vi "貪食蛇01.vi"() -> ()   [LabVIEW 2021]
uses:
  <vilib>/Utility/inputDevices.llb/keyboardAcquire.vi
  <vilib>/Utility/inputDevices.llb/closeKeyboard.vi
panel:
  out "第三次果實":dbl
  out "第二次果實":dbl
  out "第一次果實":dbl
  out "達成成就":string
  in  "OK Button":bool
  out "String":string
  in  "reset":bool
  out "時間(秒)":dbl
  out "計分板":dbl
  in  "stop":bool
  out "Array":bool[][](array[boolean])
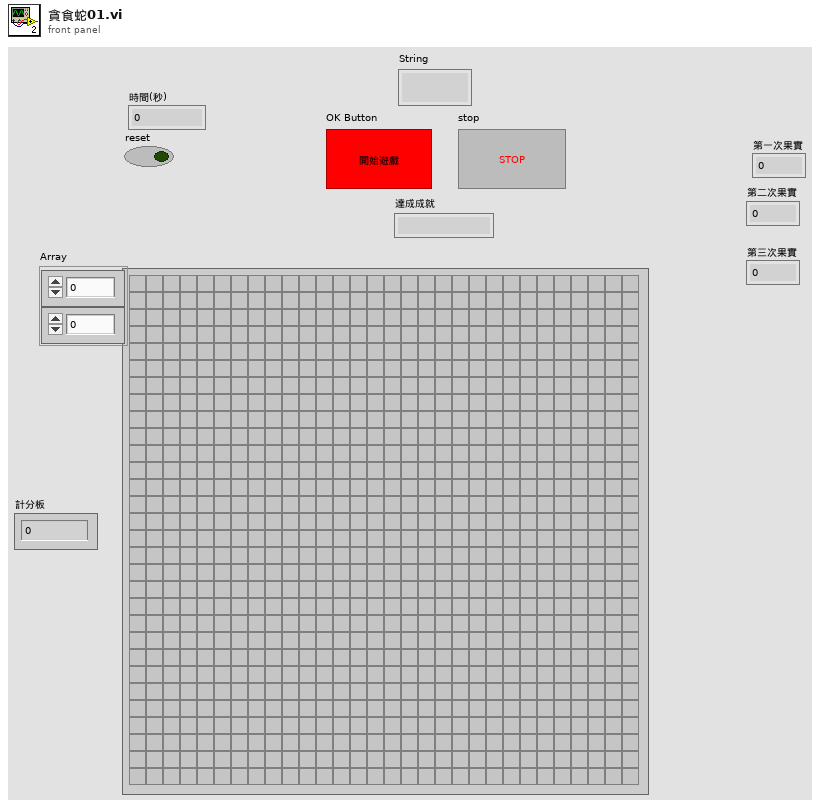
[diagram p1: front panel]
types:
  T1 = enum16{"0", "1", "2", "3", "4", "5", "6", "7", "8", "9", "A", "B", "C", "D", "E", "F", "G", "H", "I", "J", "K", "L", "M", "N", "O", "P", "Q", "R", "S", "T", "U", "V", "W", "X", "Y", "Z", "F1", "F2", "F3", "F4", "F5", "F6", "F7", "F8", "F9", "F10", "F11", "F12", "F13", "F14", "F15", "ADD", "BACK", "BACKSLASH", "CAPITAL", "COMMA", "DECIMAL", "DELETE", "DIVIDE", "DOWN", "END", "EQUALS", "ESCAPE", "GRAVE (`)", "HOME", "INSERT", "LBRACKET", "LCONTROL", "LEFT", "L ALT", "LSHIFT", "LWIN", "MINUS", "MULTIPLY", "NEXT", "NUMLOCK", "NUMPAD_0", "NUMPAD_1", "NUMPAD_2", "NUMPAD_3", "NUMPAD_4", "NUMPAD_5", "NUMPAD_6", "NUMPAD_7", "NUMPAD_8", "NUMPAD_9", "PAUSE", "PERIOD", "PRIOR (PG UP)", "RBRACKET", "RCONTROL", "RETURN", "RIGHT", "R ALT", "RSHIFT", "RWIN", "SCROLL", "SEMICOLON", "SLASH", "SPACE", "SUBTRACT", "TAB", "UP", "ENTER (num pad)", "' (quote)"}[]
  T2 = enum16{"0", "1", "2", "3", "4", "5", "6", "7", "8", "9", "A", "B", "C", "D", "E", "F", "G", "H", "I", "J", "K", "L", "M", "N", "O", "P", "Q", "R", "S", "T", "U", "V", "W", "X", "Y", "Z", "F1", "F2", "F3", "F4", "F5", "F6", "F7", "F8", "F9", "F10", "F11", "F12", "F13", "F14", "F15", "ADD", "BACK", "BACKSLASH", "CAPITAL", "COMMA", "DECIMAL", "DELETE", "DIVIDE", "DOWN", "END", "EQUALS", "ESCAPE", "GRAVE (`)", "HOME", "INSERT", "LBRACKET", "LCONTROL", "LEFT", "L ALT", "LSHIFT", "LWIN", "MINUS", "MULTIPLY", "NEXT", "NUMLOCK", "NUMPAD_0", "NUMPAD_1", "NUMPAD_2", "NUMPAD_3", "NUMPAD_4", "NUMPAD_5", "NUMPAD_6", "NUMPAD_7", "NUMPAD_8", "NUMPAD_9", "PAUSE", "PERIOD", "PRIOR (PG UP)", "RBRACKET", "RCONTROL", "RETURN", "RIGHT", "R ALT", "RSHIFT", "RWIN", "SCROLL", "SEMICOLON", "SLASH", "SPACE", "SUBTRACT", "TAB", "UP", "ENTER (num pad)", "' (quote)"}
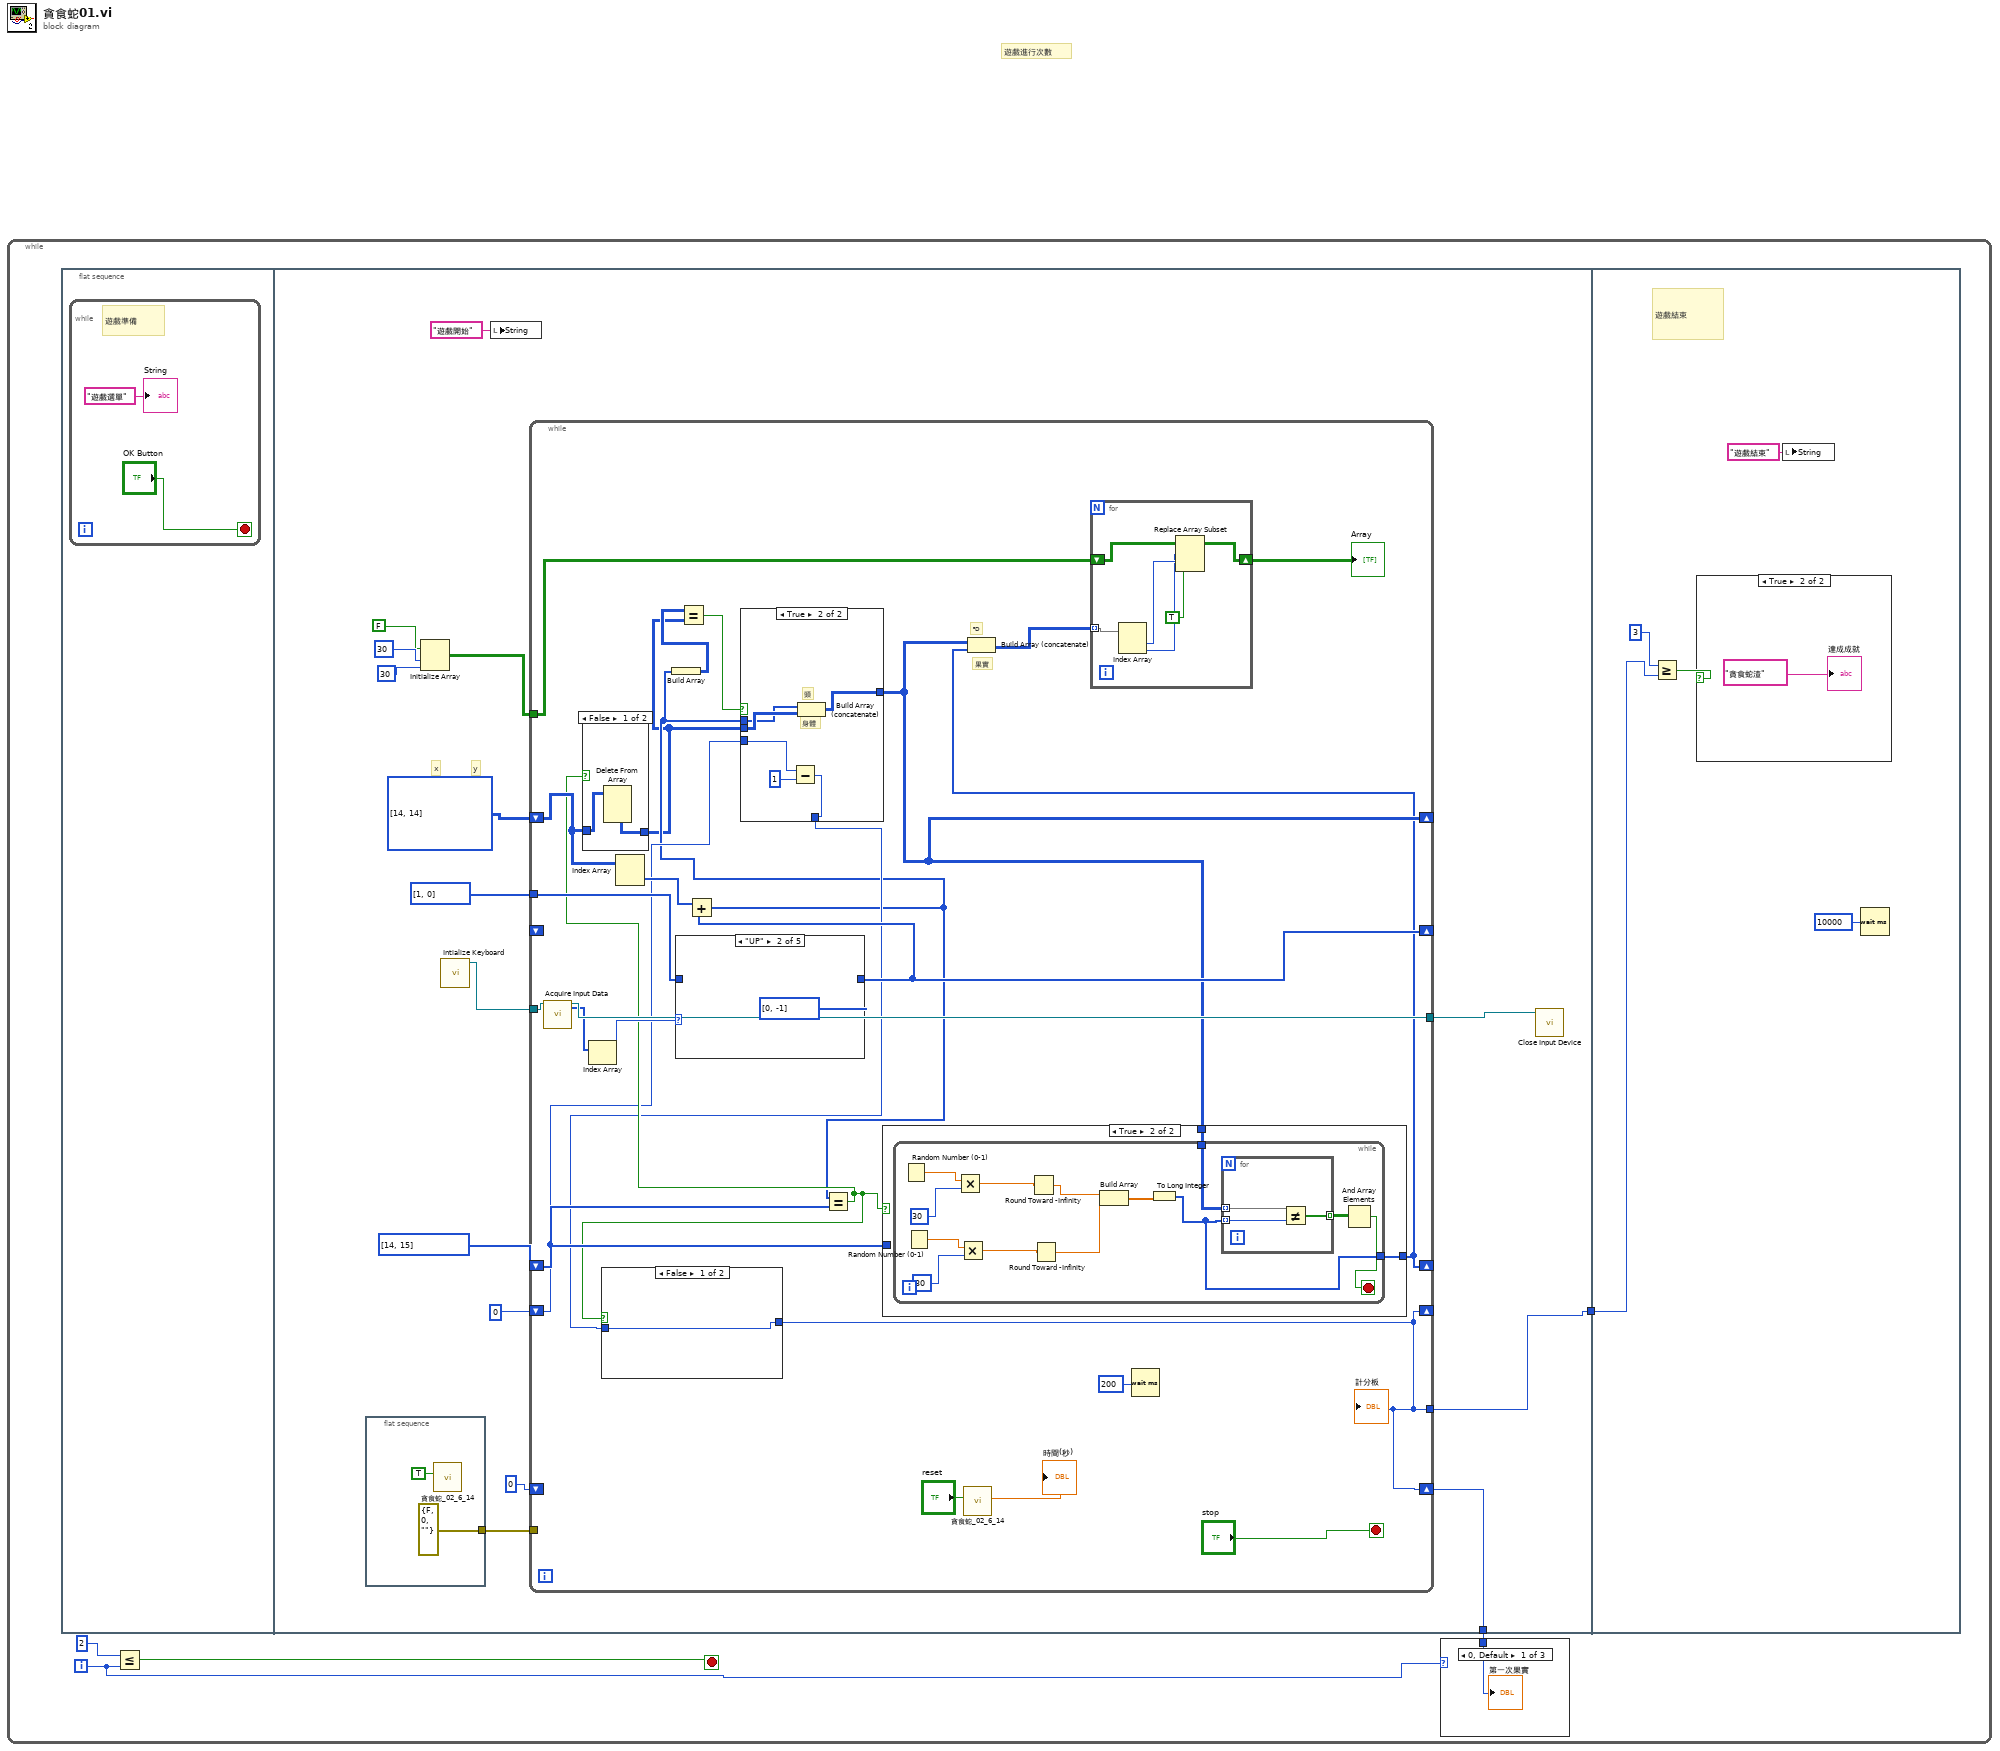
[diagram p0: block diagram]
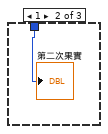
[diagram p2: hidden frame]
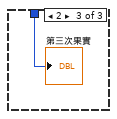
[diagram p3: hidden frame]
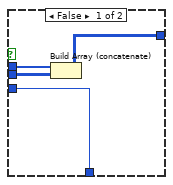
[diagram p4: hidden frame]
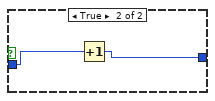
[diagram p5: hidden frame]
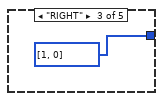
[diagram p9: hidden frame]
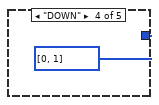
[diagram p10: hidden frame]
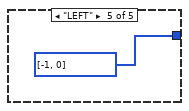
[diagram p11: hidden frame]
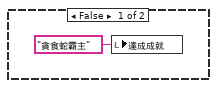
[diagram p12: hidden frame]
diagram:
  # "遊戲進行次數"
  n1 = while {
    i -> [w2]
    stop <- w3 stop-if-true
    n2 = flat-sequence {
      tunnel: [w13] -> w5
      tunnel: [w11] -> w1
      tunnel: w5 -> [w102]
      frame #0 {
        n3 = while {
          stop <- "OK Button" stop-if-true
          # "遊戲準備"
          "String" <- "遊戲選單" ("String")
        }
      }
      frame #1 {
        # "y"
        # "x"
        n4 = flat-sequence {
          tunnel: [errorcluster {"status"=FALSE, "code"=0, "source"=""} ("error constant")] -> w15
          frame #0 {
            n5 = call "貪食蛇_02_6_14.vi"("reset"=TRUE) -> ()  [unwired: 10 in, 1 out]
          }
        }
        n6 = Initialize Array(FALSE, 30, 30) -> (w22:bool[][])
        n7 = call <vilib>:"Intialize Keyboard.vi"() -> ("device ID"=w21:refnum<k1>)  [unwired: 10 in, 1 out]
        n8 = local write "String"("遊戲開始" ("String")) -> ()
        n9 = while {
          tunnel: w22 -> [w50]
          tunnel: w21 -> [w52]
          tunnel: [w51] -> w20
          shift-right: [w43] -> _
          shift-left: i32[][] [[14, 14]] -> [w44]
          shift-right: [w45] -> _
          shift-left: _ -> [_]
          tunnel: i32[] [1, 0] -> [w47]
          shift-right: [w40] -> _
          shift-left: i32[] [14, 15] -> [w42]
          shift-right: [w34] -> _
          shift-left: 0 -> [w33]
          tunnel: w15 -> [_]
          tunnel: [w34] -> w13
          shift-right: [w34] -> w11
          shift-left: 0 -> [_]
          stop <- "stop" stop-if-true
          # "果實"
          # "³D"
          n10 = call-poly <vilib>:"Acquire Input Data.vi"("device ID"=w52) -> ("device ID"=w51:refnum<k1>, "keys pressed"=w37:T1)  [unwired: 16 in, 1 out]
          n11 = Index Array(array=w37) -> (element=w48:T2)  [unwired: 1 in]
          n12 = Index Array(array=w44) -> (element=w46:i32[])  [unwired: 2 in]
          n13 = case shown="\"UP\"" w48 {
            tunnel: w47 -> [w89 _ _ _ _]
            tunnel: [w89 i32[] [0, -1] i32[] [1, 0] i32[] [0, 1] i32[] [-1, 0]] -> w45
            frame "0", Default {
            }
            frame "UP" {
            }
            frame "RIGHT" {
            }
            frame "DOWN" {
            }
            frame "LEFT" {
            }
          }
          n14 = Add(x=w46, y=w45) -> (x+y=w30:i32[])
          n15 = Build Array(w30) -> (w29:i32[][])
          n16 = Equal?(x=w30, y=w42) -> (x = y?=w39:bool)
          n17 = case shown="False" w39 {
            tunnel: [w87 w88] -> w28
            tunnel: w44 -> [w86 w88]
            frame False {
              n18 = Delete From Array(array=w86) -> (array with subset deleted=w87:i32[][])  [unwired: 3 in, 1 out]
            }
            frame True {
            }
          }
          n19 = Equal?(x=w29, y=w28) -> (x = y?=w31:bool)
          n20 = case shown="True" w31 {
            tunnel: [w57 w61] -> w43
            tunnel: w30 -> [w56 w62]
            tunnel: w28 -> [w55 w63]
            tunnel: w33 -> [w54 w59]
            tunnel: [w54 w58] -> w32
            frame False {
              n21 = Build Array (concatenate)(w56, w55) -> (w57:i32[][])
            }
            frame True {
              # "身體"
              # "頭"
              n22 = Subtract(x=w59, y=1) -> (x-y=w58:i32)
              n23 = Build Array (concatenate)(w62, w63) -> (w61:i32[][])
            }
          }
          n24 = case shown="False" w39 {
            tunnel: w32 -> [w64 w66]
            tunnel: [w64 w65] -> w34
            frame False {
            }
            frame True {
              n25 = Increment(x=w66) -> (x+1=w65:i32)
            }
          }
          "計分板" <- w34
          n26 = case shown="True" w39 {
            tunnel: w43 -> [_ w69]
            tunnel: [w67 w68] -> w40
            tunnel: w42 -> [w67 _]
            frame False {
            }
            frame True {
              n27 = while {
                tunnel: w69 -> [w73]
                tunnel: [w70] -> w68
                stop <- w71 stop-if-true
                n28 = Random Number (0-1)() -> (number: 0 to 1=w82:dbl)
                n29 = Random Number (0-1)() -> (number: 0 to 1=w79:dbl)
                n30 = Multiply(x=w82, y=30) -> (x*y=w80:dbl)
                n31 = Multiply(x=w79, y=30) -> (x*y=w77:dbl)
                n32 = Round Toward -Infinity(1:w80) -> (0:w75:dbl)
                n33 = Round Toward -Infinity(1:w77) -> (0:w76:dbl)
                n34 = Build Array(w75, w76) -> (w74:dbl[])
                n35 = To Long Integer(number=w74) -> (32bit integer=w70:i32[])
                n36 = for {
                  tunnel: w70 -> [w84] mode=indexing
                  tunnel: w73 -> [w85] mode=indexing
                  tunnel: [w83] -> w72 mode=indexing
                  n37 = Not Equal?(x=w85, y=w84) -> (x != y?=w83:bool[])
                }
                n38 = And Array Elements(Boolean array=w72) -> (logical AND=w71:bool)
              }
            }
          }
          n39 = call "貪食蛇_02_6_14.vi"("reset"="reset") -> ("時間(秒)"=→"時間(秒)":dbl)  [unwired: 10 in]
          n40 = Build Array (concatenate)(w43, w40) -> (w41:i32[][])
          n41 = for {
            shift-right: [w98] -> w49
            shift-left: w50 -> [w96]
            tunnel: w41 -> [w99] mode=indexing
            n42 = Index Array(array=w99) -> (element #1=w95:i32, element #2=w94:i32)  [unwired: 2 in]
            n43 = Replace Array Subset(array=w96, new element=TRUE, index (row)=w94, index (col)=w95) -> (w98:bool[][])
          }
          "Array" <- w49
          n44 = Wait (ms)(milliseconds to wait=200) -> ()  [unwired: 1 out]
        }
        n45 = call-poly <vilib>:"Close Input Device.vi"("device ID"=w20) -> ()  [unwired: 9 in, 1 out]
      }
      frame #2 {
        # "遊戲結束"
        n46 = Greater Or Equal?(x=3, y=w102) -> (x >= y?=w103:bool)
        n47 = case shown="True" w103 {
          frame False {
            n48 = local write "達成成就"("貪食蛇霸主" ("達成成就")) -> ()
          }
          frame True {
            "達成成就" <- "貪食蛇渣" ("達成成就")
          }
        }
        n49 = local write "String"("遊戲結束" ("String")) -> ()
        n50 = Wait (ms)(milliseconds to wait=u32 10000) -> ()  [unwired: 1 out]
      }
    }
    n51 = Less Or Equal?(x=2, y=w2) -> (x <= y?=w3:bool)
    n52 = case shown="0, Default" w2 {
      tunnel: w1 -> [w6 w7 w8]
      frame 0, Default {
        "第一次果實" <- w6
      }
      frame 1 {
        "第二次果實" <- w7
      }
      frame 2 {
        "第三次果實" <- w8
      }
    }
  }
